vi "Configure Waveform Modulation.vi"   [LabVIEW 2010, in "Agilent 2000 3000 X-Series.lvlib"]
doc: "Configures waveform modulation."
uses:
  <instrlib>/Agilent 2000 3000 X-Series/Agilent 2000 3000 X-Series.lvlib
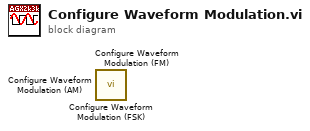
[diagram p0: block diagram]
diagram:
  n1 = call <instrlib>:"Configure Waveform Modulation (FSK).vi"() -> ()  [unwired: 10 in, 2 out]
  n2 = call <instrlib>:"Configure Waveform Modulation (FM).vi"() -> ()  [unwired: 10 in, 2 out]
  n3 = call <instrlib>:"Configure Waveform Modulation (AM).vi"() -> ()  [unwired: 10 in, 2 out]
